vi "StellarNet Set Default C-Coefficients.vi"(11 "Channel (1-based)":u8) -> (3 "Coefficients":ext[](array[numeric]))   [LabVIEW 2023]
panel:
  in  "Array":T1(array[cluster])=[{"Default Value"=0.718, "Description"="C1"}, {"Default Value"=0.00062, "Description"="C2"}, {"Default Value"=200.0, "Description"="C3"}, {"Default Value"=0.0, "Description"="C4"}]
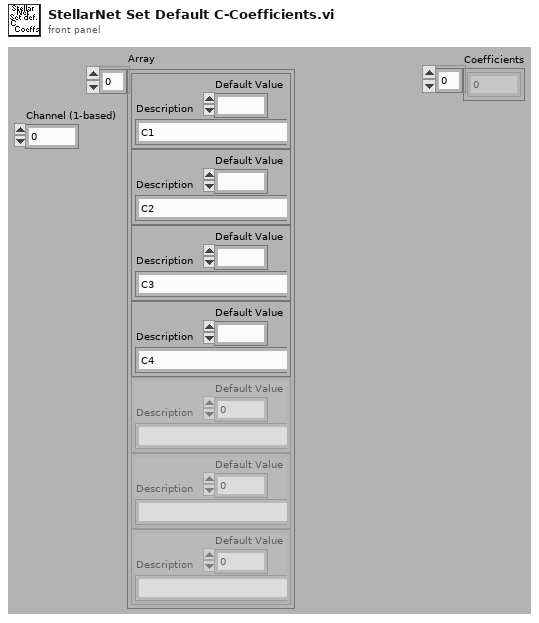
[diagram p1: front panel]
types:
  T1 = cluster{"Default Value":ext, "Description":string}[]
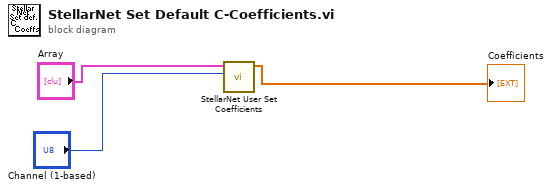
[diagram p0: block diagram]
diagram:
  n1 = call "StellarNet User Set Coefficients.vi"("Channel"="Channel (1-based)", "Array"="Array") -> ("Coeffs"=→"Coefficients":dbl[])  [unwired: 9 in]
